vi "GPIB_Trigger.vi"(2 "error in":errorcluster, 3 "address string":string) -> (0 "error out":errorcluster, 1 "status":bool[](array[boolean]))   [LabVIEW 2010]
uses:
  Controls/GPIB_Mode.ctl
  Globals/Dynamic_call_global.ph.vi
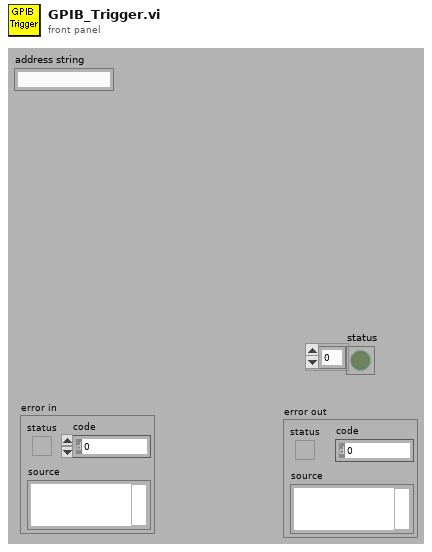
[diagram p1: front panel]
types:
  T1 = typedef "GPIB_Mode.ctl" = enum16{"Read", "Write", "Trigger", "Poll"}
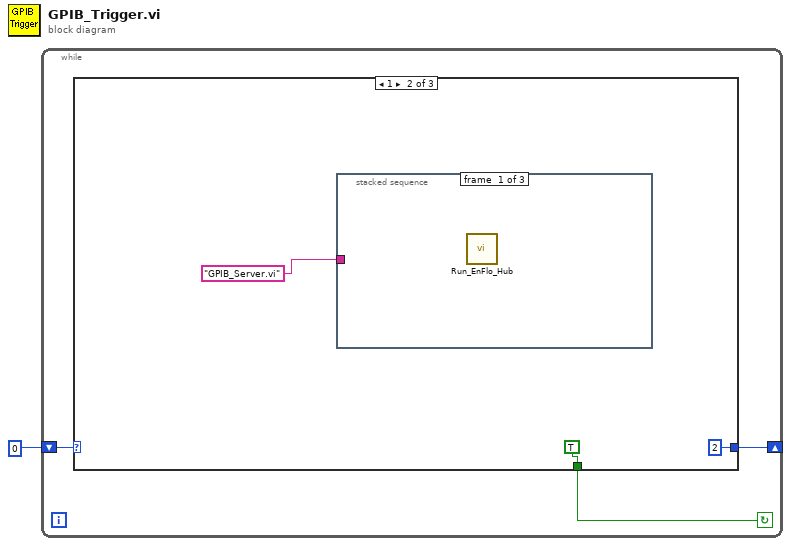
[diagram p0: block diagram]
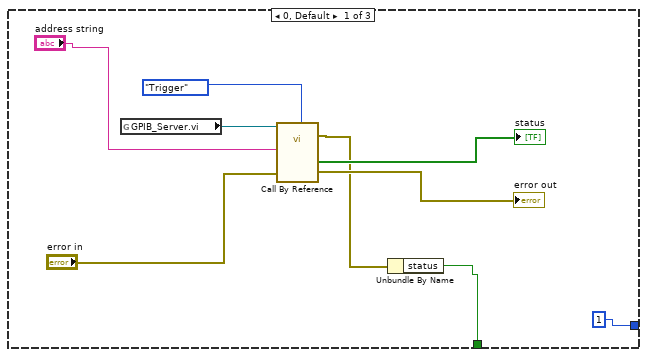
[diagram p2: hidden frame]
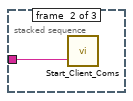
[diagram p3: hidden frame]
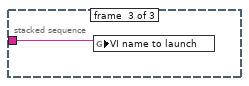
[diagram p4: hidden frame]
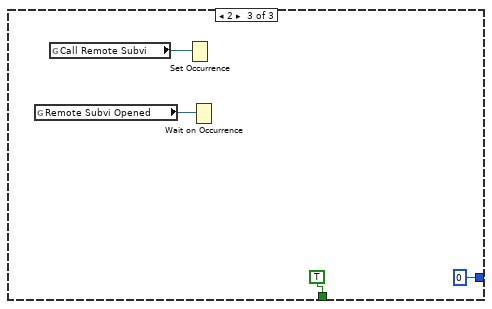
[diagram p5: hidden frame]
diagram:
  n1 = while {
    shift-right: [w3] -> _
    shift-left: 0 -> [w4]
    stop <- w2 continue-if-true
    n2 = case shown="1" w4 {
      tunnel: [1 2 0] -> w3
      tunnel: [w5 TRUE ("status") TRUE ("status")] -> w2
      frame 0, Default {
        n3 = global read "Dynamic_call_global.ph.vi" "GPIB_Server.vi"() -> (w13:refnum<vi>)
        n4 = call-by-ref "?"(reference=w13, "Case"=GPIB_Mode."Trigger", "error in"="error in", "address string"="address string") -> (error out=w7:errorcluster, 0:"error out"=→"error out":errorcluster, "status"=→"status":bool[])  [unwired: 6 in, 2 out]
        n5 = Unbundle By Name(w7) -> ("status"=w5:bool)
      }
      frame 1 {
        n6 = stacked-sequence {
          tunnel: "GPIB_Server.vi" ("VI name to launch") -> [_ w17 w18]
          frame #0 {
            n7 = call "Run_EnFlo_Hub.vi"() -> ()  [unwired: 8 out]
          }
          frame #1 {
            n8 = call "Start_Client_Coms.vi"("VI name to run on server"=w17) -> ()  [unwired: 1 in, 4 out]
          }
          frame #2 {
            n9 = global write "Dynamic_call_global.ph.vi" "VI name to launch"(w18) -> ()
          }
        }
      }
      frame 2 {
        n10 = global read "Dynamic_call_global.ph.vi" "Remote Subvi Opened"() -> (w21:refnum<k4>)
        n11 = global read "Dynamic_call_global.ph.vi" "Call Remote Subvi"() -> (w22:refnum<k4>)
        n12 = Set Occurrence(w22) -> ()
        n13 = Wait on Occurrence(2:w21) -> ()  [unwired: 3 out]
      }
    }
  }
